vi "Write Boolean.vi"(8 "error in (no error)":errorcluster, 9 "Boolean":bool=TRUE, 10 "Label":string, 11 "FlexWorktable in":refnum<class "FlexWorktable.lvclass">) -> (0 "error out":errorcluster, 3 "FlexWorktable out":refnum<class "FlexWorktable.lvclass">)   [LabVIEW 2017, in "FlexWorktable.lvclass"]
uses:
  FlexWorktable.lvclass
  FlexWorktable.lvclass/FlexWorktable.ctl
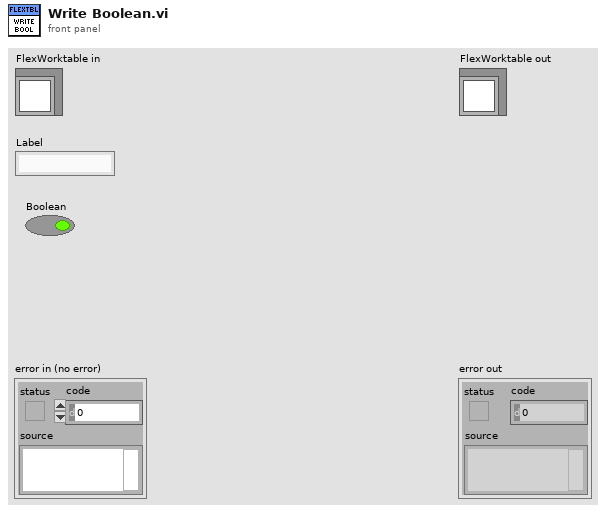
[diagram p1: front panel]
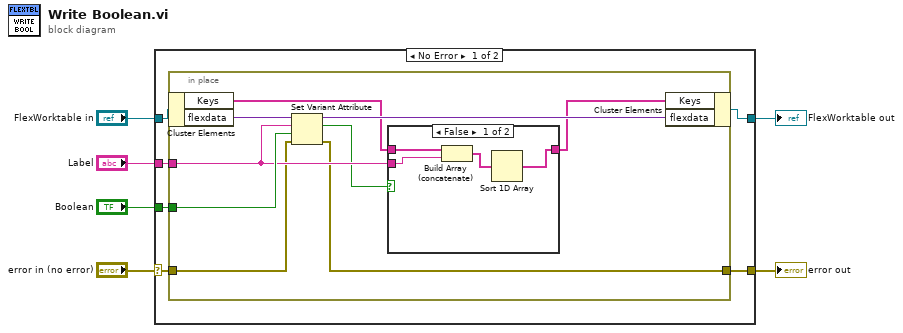
[diagram p0: block diagram]
diagram:
  n1 = case shown="No Error" "error in (no error)" {
    selector: "error in (no error)" -> [w11 w28]
    tunnel: [w8 w28] -> w5
    tunnel: [w7 w27] -> w3
    tunnel: "FlexWorktable in" -> [w12 w27]
    tunnel: "Label" -> [w10 _]
    tunnel: "Boolean" -> [w9 _]
    frame No Error {
      n2 = in-place {
        in-place-border: w11 -> [w16]
        in-place-border: w10 -> [w17]
        in-place-border: w9 -> [w20]
        in-place-border: [w15] -> w8
        n3 = in-place-cluster #1(w12) -> ("Keys"=w18:string[], "flexdata"=w21:variant)
        n4 = Set Variant Attribute(Variant=w21, name=w17, value=w20, error in=w16) -> (Variant out=w19:variant, replaced=w14:bool, error out=w15:errorcluster)
        n5 = case shown="False" w14 {
          tunnel: w18 -> [w25 w26]
          tunnel: w17 -> [w24 _]
          tunnel: [w22 w26] -> w13
          frame False {
            n6 = Build Array (concatenate)(w25, w24) -> (w23:string[])
            n7 = Sort 1D Array(array=w23) -> (sorted array=w22:string[])
          }
          frame True {
          }
        }
        n8 = in-place-cluster #1("Keys"=w13, "flexdata"=w19) -> (w7:refnum<class "FlexWorktable.lvclass">)
      }
    }
    frame Error {
    }
  }
  "error out" <- w5
  "FlexWorktable out" <- w3
